vi "Exercice 1 4 opérations.vi"() -> ()   [LabVIEW 2018]
panel:
  out "Numeric 12":dbl format="%#.3g"
  in  "Numeric 11":dbl
  in  "Numeric 10":dbl
  out "Numeric 9":dbl
  in  "Numeric 8":dbl
  in  "Numeric 7":dbl
  out "Numeric 6":dbl
  in  "Numeric 5":dbl min=0.0 max=9.0
  in  "Numeric 4":dbl min=0.0 max=9.0
  out "Numeric 3":dbl
  in  "Numeric 2":dbl min=0.0 max=9.0
  in  "Numeric":dbl min=0.0 max=9.0
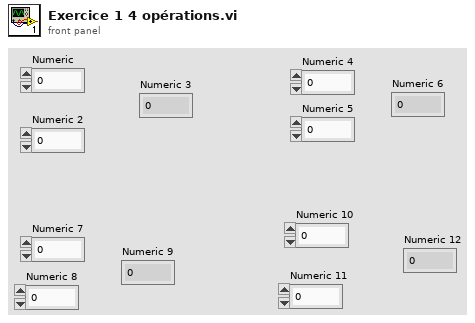
[diagram p1: front panel]
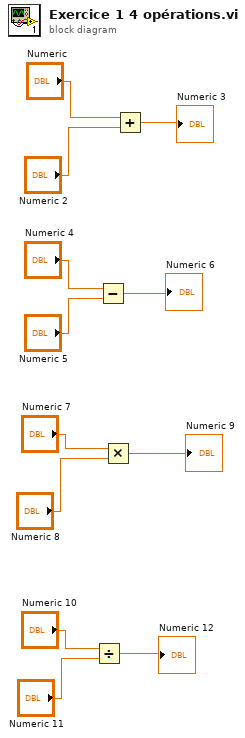
[diagram p0: block diagram]
diagram:
  n1 = Divide(x="Numeric 10", y="Numeric 11") -> (x/y=→"Numeric 12":dbl)
  n2 = Subtract(x="Numeric 4", y="Numeric 5") -> (x-y=→"Numeric 6":dbl)
  n3 = Multiply(x="Numeric 7", y="Numeric 8") -> (x*y=→"Numeric 9":dbl)
  n4 = Add(x="Numeric", y="Numeric 2") -> (x+y=→"Numeric 3":dbl)
